vi "Read Hand Position Velocity.vi"   [LabVIEW 2011, in "LMH-Leap.lvlib"]
doc: "Read the position and velocity of hand objects in the frame. Use the polymorphic instance to select one hand or N hands."
uses:
  LMH-Leap.lvlib
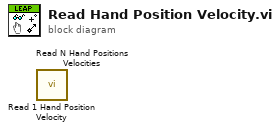
[diagram p0: block diagram]
diagram:
  n1 = call "Read 1 Hand Position Velocity.vi"() -> ()  [unwired: 8 in, 4 out]
  n2 = call "Read N Hand Positions Velocities.vi"() -> ()  [unwired: 8 in, 4 out]
